vi "OuterWorksDataWire.vi"(11 "String":string) -> (3 "result":string="N/A")   [LabVIEW 2015]
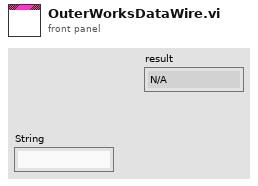
[diagram p1: front panel]
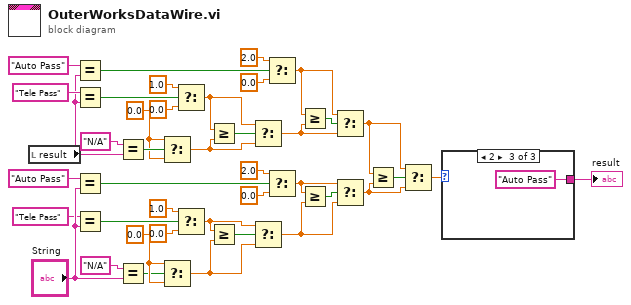
[diagram p0: block diagram]
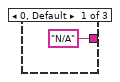
[diagram p2: hidden frame]
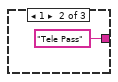
[diagram p3: hidden frame]
diagram:
  w30 = 0.0 ("t")
  w9 = 0.0 ("t")
  n1 = local read "result"() -> (w1:string)
  n2 = Equal?(x="Auto Pass", y=w1) -> (x = y?=w32:bool)
  n3 = Equal?(x="Tele Pass", y=w1) -> (x = y?=w33:bool)
  n4 = Equal?(x="Auto Pass", y="String") -> (x = y?=w6:bool)
  n5 = Equal?(x="Tele Pass", y="String") -> (x = y?=w5:bool)
  n6 = Equal?(x="N/A", y=w1) -> (x = y?=w36:bool)
  n7 = Equal?(x="N/A", y="String") -> (x = y?=w2:bool)
  n8 = Select(t=w30, s=w36, f=w30) -> (s? t:f=w23:dbl)
  n9 = Select(t=w9, s=w2, f=w9) -> (s? t:f=w16:dbl)
  n10 = Select(t=1.0, s=w33, f=0.0) -> (s? t:f=w24:dbl)
  n11 = Select(t=1.0, s=w5, f=0.0) -> (s? t:f=w15:dbl)
  n12 = Greater Or Equal?(x=w24, y=w23) -> (x >= y?=w25:bool)
  n13 = Greater Or Equal?(x=w15, y=w16) -> (x >= y?=w14:bool)
  n14 = Select(t=w24, s=w25, f=w23) -> (s? t:f=w20:dbl)
  n15 = Select(t=w15, s=w14, f=w16) -> (s? t:f=w19:dbl)
  n16 = Select(t=2.0, s=w32, f=0.0) -> (s? t:f=w21:dbl)
  n17 = Select(t=2.0, s=w6, f=0.0) -> (s? t:f=w18:dbl)
  n18 = Greater Or Equal?(x=w21, y=w20) -> (x >= y?=w22:bool)
  n19 = Greater Or Equal?(x=w18, y=w19) -> (x >= y?=w17:bool)
  n20 = Select(t=w21, s=w22, f=w20) -> (s? t:f=w39:dbl)
  n21 = Select(t=w18, s=w17, f=w19) -> (s? t:f=w40:dbl)
  n22 = Greater Or Equal?(x=w39, y=w40) -> (x >= y?=w37:bool)
  n23 = Select(t=w39, s=w37, f=w40) -> (s? t:f=w38:dbl)
  n24 = case shown="2" w38 {
    tunnel: ["N/A" ("x") "Tele Pass" ("x") "Auto Pass" ("x")] -> w41
    frame 0, Default {
    }
    frame 1 {
    }
    frame 2 {
    }
  }
  "result" <- w41
